vi "Configure Limit Line Advanced.vi"(5 "Statistics Threshold Value (0 percentage)":dbl, 6 "Enable Statistics Threshold (F: Disable)":bool, 7 "Margin (0 dB)":dbl, 8 "error in (no error)":errorcluster, 9 "Enable Margin (F: Disable)":bool, 10 "Line Number (1: Line 1)":i32(ring)=1 items=["Line 1"=1, "Line 2"=2], 11 "VISA resource name":refnum<visa-resource-name>) -> (0 "error out":errorcluster, 3 "VISA resource name out":refnum<visa-resource-name>)   [LabVIEW 2022 SP3, in "Agilent N934X Series.lvlib"]
doc: "Configure the Limit line settings.\n\nNote:\nThis VI is only applicable for N9321C, N9322C, N9323C, N9324C models."
uses:
  <instrlib>/Agilent N934X Series/Agilent N934X Series.lvlib
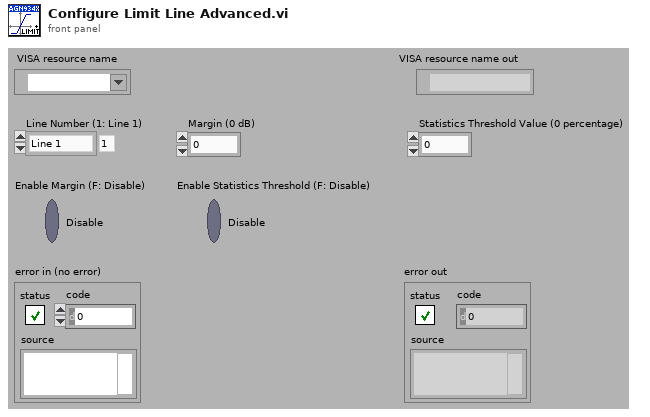
[diagram p1: front panel]
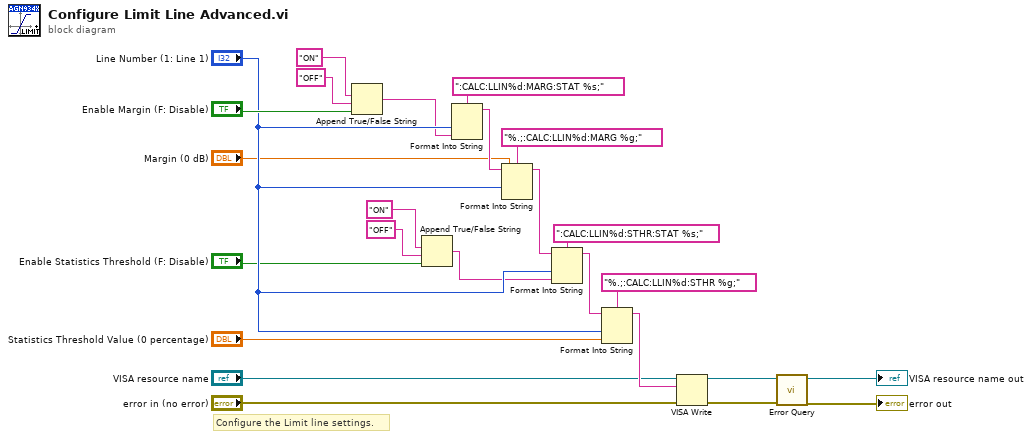
[diagram p0: block diagram]
diagram:
  # "Configure the Limit line settings."
  n1 = Append True/False String(1:"Enable Margin (F: Disable)", 2:"OFF", 3:"ON") -> (0:w20:string)  [unwired: 1 in]
  n2 = Append True/False String(1:"Enable Statistics Threshold (F: Disable)", 2:"OFF", 3:"ON") -> (0:w11:string)  [unwired: 1 in]
  n3 = Format Into String(format string=":CALC:LLIN%d:MARG:STAT %s;", "Line Number (1: Line 1)", w20) -> (resulting string=w19:string)  [unwired: 2 in, 1 out]
  n4 = Format Into String(format string="%.;:CALC:LLIN%d:MARG %g;", initial string=w19, "Line Number (1: Line 1)", "Margin (0 dB)") -> (resulting string=w13:string)  [unwired: 1 in, 1 out]
  n5 = Format Into String(format string=":CALC:LLIN%d:STHR:STAT %s;", initial string=w13, "Line Number (1: Line 1)", w11) -> (resulting string=w10:string)  [unwired: 1 in, 1 out]
  n6 = Format Into String(format string="%.;:CALC:LLIN%d:STHR %g;", initial string=w10, "Line Number (1: Line 1)", "Statistics Threshold Value (0 percentage)") -> (resulting string=w7:string)  [unwired: 1 in, 1 out]
  n7 = VISA Write(VISA resource name="VISA resource name", write buffer=w7, error in (no error)="error in (no error)") -> (VISA resource name out=w4:refnum<visa-resource-name>, error out=w3:errorcluster)  [unwired: 1 out]
  n8 = call <instrlib>:"Error Query.vi"("error in (no error)"=w3, "VISA resource name"=w4) -> ("error out"=→"error out":errorcluster, "VISA resource name out"=→"VISA resource name out":refnum<visa-resource-name>)  [unwired: 6 in, 2 out]
